vi "Clear Specific Errors.vi"(8 "Error In":errorcluster, 11 "Error number In":i32) -> (0 "Error Out":errorcluster, 3 "Error Cleared?":bool)   [LabVIEW 2017]
doc: "SciScan 1.2 160622\nThis is a modified version of the clear errors function provided by labview.\nThe error# that needs to be cleared has to be specified by the developer"
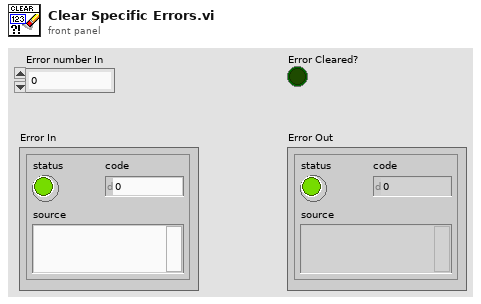
[diagram p1: front panel]
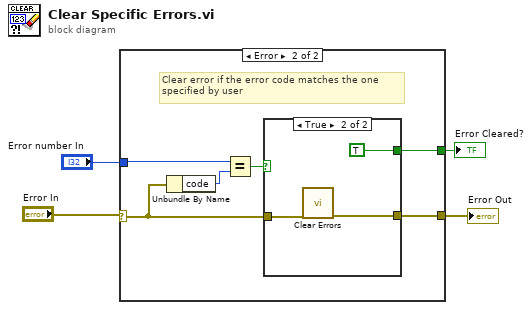
[diagram p0: block diagram]
diagram:
  n1 = case shown="Error" "Error In" {
    selector: "Error In" -> [w5 w8]
    tunnel: "Error number In" -> [_ w10]
    tunnel: [w5 w7] -> w2
    tunnel: [_ w6] -> w1
    frame No Error {
    }
    frame Error {
      # "Clear error if the error code matches the one specified by user"
      n2 = Unbundle By Name(w8) -> ("code"=w11:i32)
      n3 = Equal?(x=w10, y=w11) -> (x = y?=w9:bool)
      n4 = case shown="True" w9 {
        tunnel: w8 -> [w12 w15]
        tunnel: [w12 w14] -> w7
        tunnel: [_ TRUE] -> w6
        frame False {
        }
        frame True {
          n5 = call <vilib>:"Clear Errors.vi"("error in (no error)"=w15) -> ("error out"=w14:errorcluster)  [unwired: 5 in, 1 out]
        }
      }
    }
  }
  "Error Out" <- w2
  "Error Cleared?" <- w1
